vi "input data row.vi"(8 "error in (no error)":errorcluster, 10 "Last row of data file":string[](array[string]), 11 "Automation in":refnum<class "NMR Data.lvclass">) -> (0 "error out":errorcluster, 2 "Added new data point?":bool, 3 "Automation out":refnum<class "NMR Data.lvclass">, 4 "Pol":dbl, 6 "Event Num":i64)   [LabVIEW 2019, in "NMR Data.lvclass"]
uses:
  NMR Data.lvclass
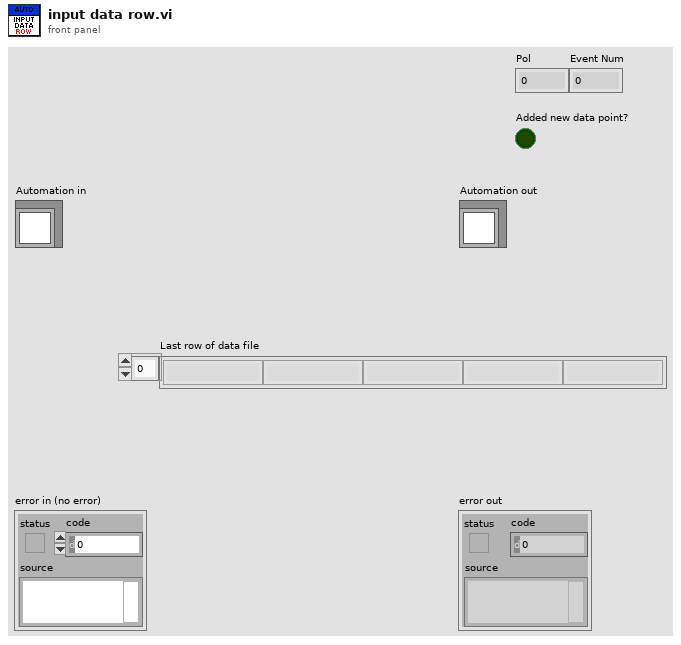
[diagram p1: front panel]
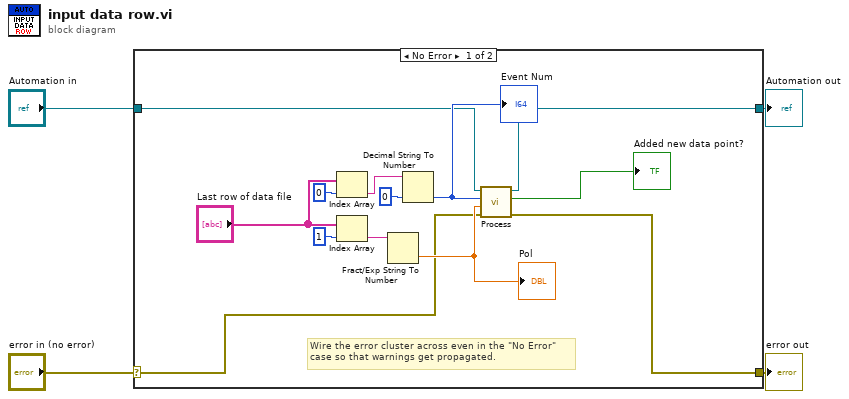
[diagram p0: block diagram]
diagram:
  n1 = case shown="No Error" "error in (no error)" {
    selector: "error in (no error)" -> [w6 w19]
    tunnel: [w7 w19] -> w3
    tunnel: [w8 w18] -> w1
    tunnel: "Automation in" -> [w9 w18]
    frame No Error {
      # "Wire the error cluster across even in the \"No Error\"\ncase so that warnings get propagated."
      n2 = Index Array(array="Last row of data file", index=0) -> (element=w15:string)
      n3 = Index Array(array="Last row of data file", index=1) -> (element=w14:string)
      n4 = Fract/Exp String To Number(string=w14) -> (number=w10:dbl)  [unwired: 3 in, 1 out]
      "Pol" <- w10
      n5 = Decimal String To Number(string=w15, default (0L)=i64 0 ("default (0 I32)")) -> (number=w11:i64)  [unwired: 1 in, 1 out]
      "Event Num" <- w11
      n6 = call "Process.vi"("error in (no error)"=w6, "New polarization"=w10, "New eventnum"=w11, "Automation in"=w9) -> ("error out"=w7:errorcluster, "Added new data point?"=→"Added new data point?":bool, "Automation out"=w8:refnum<class "NMR Data.lvclass">)  [unwired: 5 in]
    }
    frame Error {
    }
  }
  "error out" <- w3
  "Automation out" <- w1
